vi "ExternalGetParam.vi"(0 "reference in":refnum<class "VINode.lvclass">, 1 "setParameter":T2, 5 "error in (no error)":errorcluster) -> (14 "reference out":refnum<class "VINode.lvclass">, 15 "string":string, 16 "position":T1 {"y" format="%.2f"; "x" format="%.2f"}, 18 "Path":path, 19 "error out":errorcluster)   [LabVIEW 2020, in "VINode.lvclass"]
doc: "Sets parameter externaly.\nPossible to set Name,Attrib,Methods and Position"
uses:
  <resource>/Framework/Providers/Open_GDS/UML/VINode_class/VINode.lvclass
  C:/Program Files (x86)/National Instruments/LabVIEW 2020/resource/Framework/Providers/Open_GDS/UML/RectangularNode_class/RectangularNode.lvclass
  <resource>/Framework/Providers/Open_GDS/UML/VINode_class/ExternalSetTypes.ctl
  <resource>/Framework/Providers/Open_GDS/UML/General/Point/Point Point2D.ctl
  <resource>/Framework/Providers/Open_GDS/UML/MultiLineString_class/MultiLineString.lvclass
  <resource>/Framework/Providers/Open_GDS/UML/RectangularNode_class/RectangularNode.lvclass
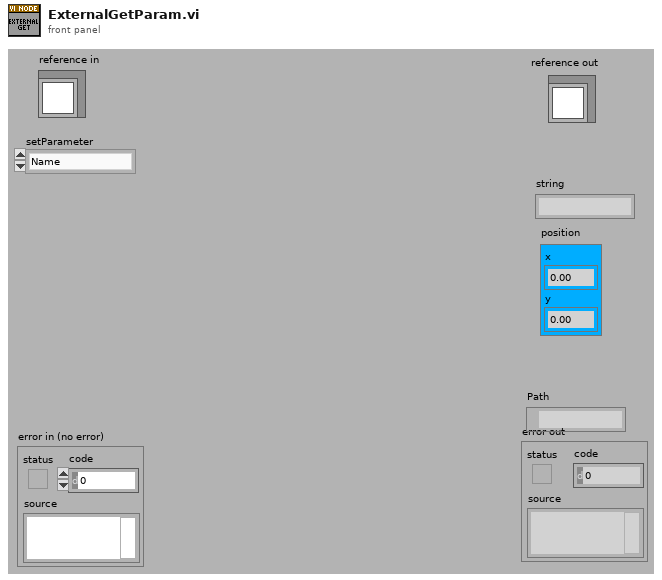
[diagram p1: front panel]
types:
  T1 = typedef "Point Point2D.ctl" = cluster{"x":dbl, "y":dbl}
  T2 = typedef "VINode.lvclass/ExternalSetTypes.ctl" = enum16{"Name", "ClassPath", "Position", "Description"}
  T3 = typedef "VINode.lvclass/ObjectAttributes.ctl" = cluster{"midHeight":dbl, "botHeight":dbl, "Name":refnum<class "MultiLineString.lvclass">, "DEFAULT_COMPARTMENT_HEIGHT":i32, "DEFAULT_WIDTH":i32, "DEFAULT_HEIGHT":i32, "VIPath":path, "Description":refnum<class "MultiLineString.lvclass">, "ShowDescription":bool}
  T4 = typedef "RectangularNode.lvclass/ObjectAttributes.ctl" = cluster{"bounds":T5}
  T5 = typedef "Rectangle Rectangle2D.ctl" = cluster{"x":dbl, "y":dbl, "width":dbl, "height":dbl}
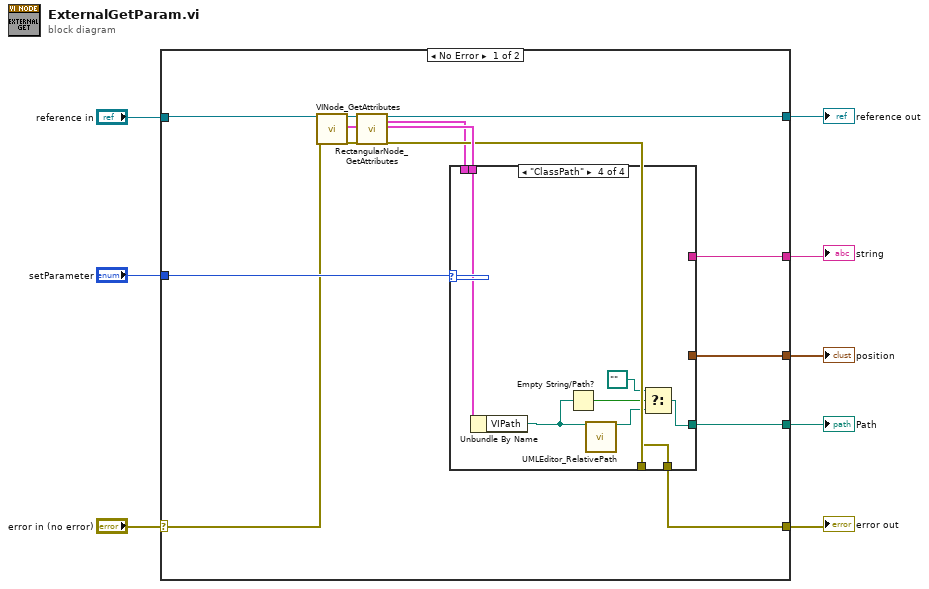
[diagram p0: block diagram]
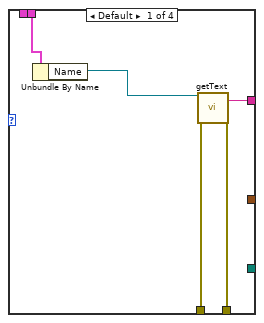
[diagram p2: hidden frame]
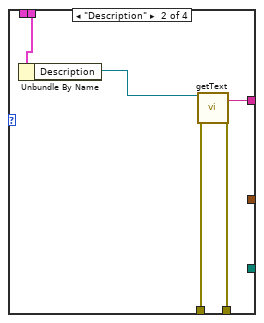
[diagram p3: hidden frame]
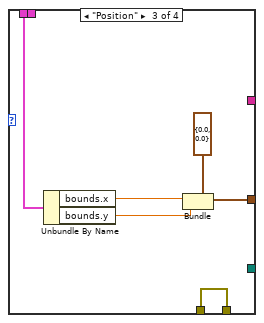
[diagram p4: hidden frame]
diagram:
  n1 = case shown="No Error" "error in (no error)" {
    selector: "error in (no error)" -> [w19 w45]
    tunnel: "reference in" -> [w21 w46]
    tunnel: [w18 w45] -> w6
    tunnel: [w10 w46] -> w5
    tunnel: "setParameter" -> [w20 _]
    tunnel: [w17 _] -> w3
    tunnel: [w16 _] -> w2
    tunnel: [w15 _] -> w1
    frame No Error {
      n2 = call <resource>:"VINode_GetAttributes.vi"("reference in"=w21, "error in (no error)"=w19) -> ("reference out"=w13:refnum<class "VINode.lvclass">, "Data"=w14:T3, "error out"=w12:errorcluster)  [unwired: 1 in, 14 out]
      n3 = call <resource>:"RectangularNode_GetAttributes.vi"("reference in"=w13, "error in (no error)"=w12) -> ("reference out"=w10:refnum<class "VINode.lvclass">, "Data"=w9:T4, "error out"=w11:errorcluster)  [unwired: 14 in, 1 out]
      n4 = case shown="\"ClassPath\"" w20 {
        tunnel: w11 -> [w26 w31 w37 w44]
        tunnel: [w25 w30 w37 w44] -> w18
        tunnel: [_ _ w33 _] -> w17
        tunnel: [w23 w28 _ _] -> w16
        tunnel: [_ _ _ w40] -> w15
        tunnel: w14 -> [w22 w27 _ w38]
        tunnel: w9 -> [_ _ w32 _]
        frame Default {
          n5 = Unbundle By Name(w22) -> ("Name"=w24:refnum<class "MultiLineString.lvclass">)
          n6 = call-dynamic "getText.vi"("reference"=w24, "error in (no error)"=w26) -> ("text"=w23:string, "error out"=w25:errorcluster)  [unwired: 16 out]
        }
        frame "Description" {
          n7 = Unbundle By Name(w27) -> ("Description"=w29:refnum<class "MultiLineString.lvclass">)
          n8 = call-dynamic "getText.vi"("reference"=w29, "error in (no error)"=w31) -> ("text"=w28:string, "error out"=w30:errorcluster)  [unwired: 16 out]
        }
        frame "Position" {
          n9 = Unbundle By Name(w32) -> ("bounds.x"=w35:dbl, "bounds.y"=w34:dbl)
          n10 = Bundle(cluster=T1 {"x"=0.0, "y"=0.0} ("position"), "x"=w35, "y"=w34) -> (w33:T1)
        }
        frame "ClassPath" {
          n11 = Unbundle By Name(w38) -> ("VIPath"=w43:path)
          n12 = Empty String/Path?(string/path=w43) -> (empty?=w42:bool)
          n13 = call <resource>:"UMLEditor_RelativePath.vi"("Path In"=w43) -> ("ConvertToAbsolutePath(If possible)"=w41:path)  [unwired: 1 in, 17 out]
          n14 = Select(t=path "", s=w42, f=w41) -> (s? t:f=w40:path)
        }
      }
    }
    frame Error {
    }
  }
  "reference out" <- w5
  "error out" <- w6
  "position" <- w3
  "string" <- w2
  "Path" <- w1
